vi "Determine State.vi"(10 "Motor In":cluster{"Port":T2, "Port":T2}={"Port"=1, "Port"=3} {"Port" items=["Port A", "Port B", "Port C", "Port D"]; "Port" items=["Port A", "Port B", "Port C", "Port D"]}, 11 "Ref in":T1) -> (1 "State":i16, 2 "Motor Out":cluster{"Port":T2, "Port":T2} {"Port" items=["Port A", "Port B", "Port C", "Port D"]; "Port" items=["Port A", "Port B", "Port C", "Port D"]}, 3 "Ref Out":T1)   [LabVIEW 2014]
doc: "Determine State \n\nFrom the 4 sensors, it calculates which \"state\" it is in.\n\nSensor Ports:\n1 - Light. 2 - Front, 3 - Left, 4 - Right\n\nStates:\nSpin : 0, 3,5,6,7,11,13,14,15\nRight Bumped: 1\nLeft Bumped: 2\nFront Bumped: 4\nOut of Bounds: 8\nOut of Bounds and Right Bumped :9 \nOut of Bounds and Left Bumped :10\nOut of Bounds and Front Bumped : 12"
uses:
  <vilib>/NXT/Subs/LVHSConnector.ctl
  <vilib>/NXT/LegoClasses/BrickReference/BrickReference.lvclass
  <vilib>/NXT/Block Support/NXT_OutputPort.ctl
  <vilib>/NXT/Block Support/NXT_InputPort.ctl
  <vilib>/NXT/Dual Mode Library/Sensors/Touch_Pressed.vi
  <vilib>/NXT/Dual Mode Library/Display/drawNumber.vi
panel:
  # "Beverly Abadines\nPhys 350\nP7"
  # "Determine State"
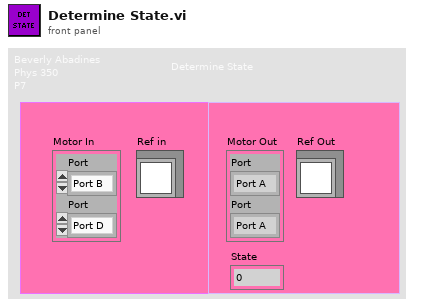
[diagram p1: front panel]
types:
  T1 = typedef "LVHSConnector.ctl" = refnum<class "BrickReference.lvclass">
  T2 = typedef "NXT_OutputPort.ctl" = u8
  T3 = typedef "NXT_InputPort.ctl" = u32
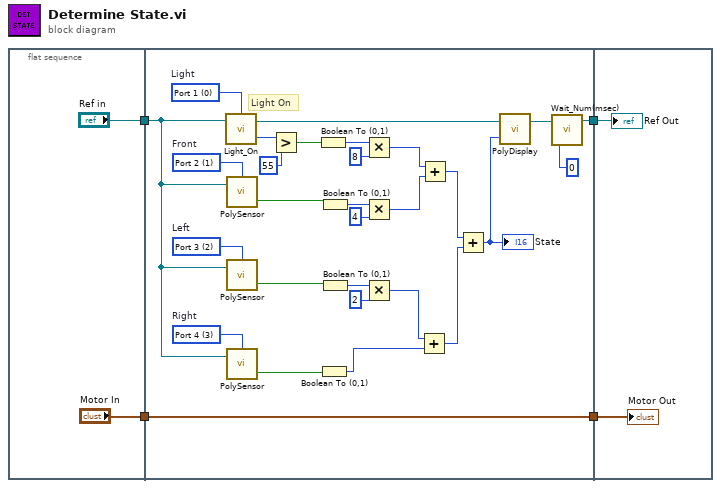
[diagram p0: block diagram]
diagram:
  n1 = flat-sequence {
    tunnel: ["Ref in"] -> w4
    tunnel: ["Motor In"] -> w1
    tunnel: w4 -> [w7]
    tunnel: [w7] -> w3
    tunnel: [w8] -> w2
    tunnel: w1 -> [w8]
    tunnel: w3 -> [w35]
    tunnel: w2 -> [w36]
    frame #0 {
    }
    frame #1 {
      w12 = T3 3 items=["Port 1", "Port 2", "Port 3", "Port 4"]  # Right
      w11 = T3 2 items=["Port 1", "Port 2", "Port 3", "Port 4"]  # Left
      w10 = T3 1 items=["Port 1", "Port 2", "Port 3", "Port 4"]  # Front
      w9 = T3 0 items=["Port 1", "Port 2", "Port 3", "Port 4"]  # Light
      # "Light On"
      n2 = call <vilib>:"Light_On.vi"("Port (Port 3)"=w9) -> ("Scaled Value"=w13:i16, "NXT/EV3"=w31:T1)  [unwired: 2 in]
      n3 = call-poly <vilib>:"PolySensor.vi"("NXT/EV3"=w7, "Port (Port 1)"=w10) -> ("Yes / No"=w16:bool)  [unwired: 1 in, 1 out]
      n4 = call-poly <vilib>:"PolySensor.vi"("NXT/EV3"=w7, "Port (Port 1)"=w11) -> ("Yes / No"=w17:bool)  [unwired: 1 in, 1 out]
      n5 = call-poly <vilib>:"PolySensor.vi"("NXT/EV3"=w7, "Port (Port 1)"=w12) -> ("Yes / No"=w18:bool)  [unwired: 1 in, 1 out]
      n6 = Greater?(x=w13, y=i16 55) -> (0:w15:bool)
      n7 = Boolean To (0,1)(Boolean=w15) -> (0, 1=w19:i16)
      n8 = Boolean To (0,1)(Boolean=w18) -> (0, 1=w28:i16)
      n9 = Boolean To (0,1)(Boolean=w16) -> (0, 1=w20:i16)
      n10 = Boolean To (0,1)(Boolean=w17) -> (0, 1=w21:i16)
      n11 = Multiply(x=w19, y=i16 8) -> (x*y=w25:i16)
      n12 = Multiply(x=w20, y=i16 4) -> (x*y=w26:i16)
      n13 = Multiply(x=w21, y=i16 2) -> (x*y=w27:i16)
      n14 = Add(x=w27, y=w28) -> (x+y=w29:i16)
      n15 = Add(x=w25, y=w26) -> (x+y=w30:i16)
      n16 = Add(x=w30, y=w29) -> (x+y=w34:i16)
      "State" <- w34
      n17 = call-poly <vilib>:"PolyDisplay.vi"("number"=w34, "NXT/EV3"=w31) -> ("NXT/EV3"=w32:T1)  [unwired: 2 in]
      n18 = call <vilib>:"Wait_Num(msec).vi"("Time (100 msec)"=u32 0, "NXT/EV3"=w32) -> ()  [unwired: 2 in, 1 out]
    }
    frame #2 {
      "Ref Out" <- w35
      "Motor Out" <- w36
    }
  }
